vi "Generator Driver Template 2.vi"() -> ()   [LabVIEW 2019]
uses:
  subVIs/Revidyne Generator.lvlib
panel:
  out "Waveform Chart":dbl(graph)
  in  "Speed":dbl(slide) scale=0.0..255.0
  in  "stop":bool
  in  "generator":refnum<visa-resource-name>
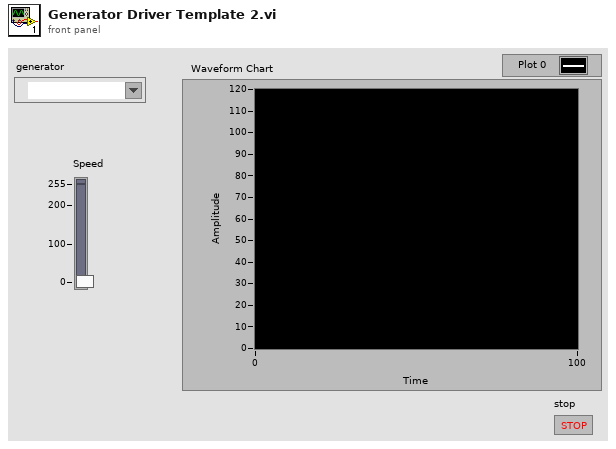
[diagram p1: front panel]
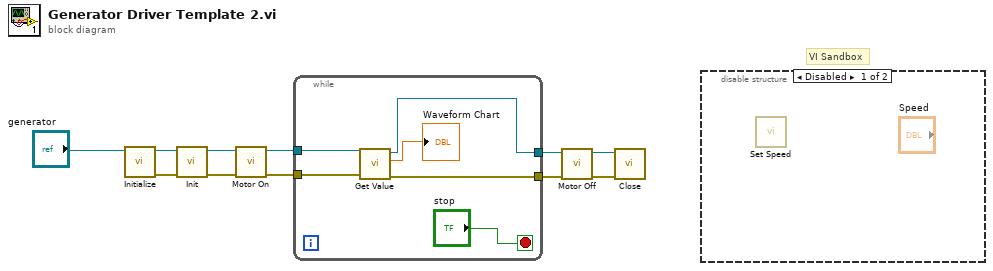
[diagram p0: block diagram]
diagram:
  # "VI Sandbox"
  n1 = call "Initialize.vi"("VISA resource name"="generator") -> ("error out"=w10:errorcluster, "VISA resource name out"=w11:refnum<visa-resource-name>)  [unwired: 9 in]
  n2 = call "Init.vi"("error in (no error)"=w10, "VISA resource name"=w11) -> ("error out"=w8:errorcluster, "VISA resource name out"=w9:refnum<visa-resource-name>)  [unwired: 8 in]
  n3 = call "Motor On.vi"("error in"=w8, "VISA resource name"=w9) -> ("error out"=w6:errorcluster, "VISA resource name out"=w7:refnum<visa-resource-name>)  [unwired: 8 in]
  n4 = while {
    tunnel: w7 -> [w17]
    tunnel: w6 -> [w16]
    tunnel: [w15] -> w5
    tunnel: [w14] -> w3
    stop <- "stop" stop-if-true
    n5 = call "Get Value.vi"("error in (no error)"=w16, "VISA resource name"=w17) -> ("error out"=w14:errorcluster, "Value"=→"Waveform Chart":dbl, "VISA resource name out"=w15:refnum<visa-resource-name>)  [unwired: 7 in]
  }
  n6 = call "Motor Off.vi"("error in (no error)"=w3, "VISA resource name"=w5) -> ("error out"=w2:errorcluster, "VISA resource name out"=w4:refnum<visa-resource-name>)  [unwired: 8 in]
  n7 = call "Close.vi"("error in (no error)"=w2, "VISA resource name"=w4) -> ()  [unwired: 9 in, 1 out]
  n8 = disable-structure shown="Disabled" {
    frame Disabled {
      n9 = call "Set Speed.vi"() -> ()  [unwired: 10 in, 2 out]
    }
    frame Enabled {
    }
  }
